vi "_시리얼_Mark10-제어 (압력설정).vi"(3 "FTS 제어 상태":T1="압력제어 시작", 4 "압력 설정(lb)":dbl=10.0 min=0.0 max=160.0 step=0.01 format="%.2f", 5 "시리얼 포트":refnum<visa-resource-name>="COM5") -> (0 "게이지 압력(lb)":dbl min=0.0 max=160.0 step=0.01 format="%.2f", 1 "통신 정상":bool=TRUE, 2 "시리얼 포트out":refnum<visa-resource-name>="COM5")   [LabVIEW 2015]
panel:
  out "미세조정 횟수":u32
  in  "속도-미세조정(mm/min)":dbl=1.0
  in  "속도-저속(mm/min)":dbl=4.0
  in  "속도-중속(mm/min)":dbl=60.0
  in  "속도-고속(mm/min)":dbl=250.0
  # "MARK10 압력 제어"
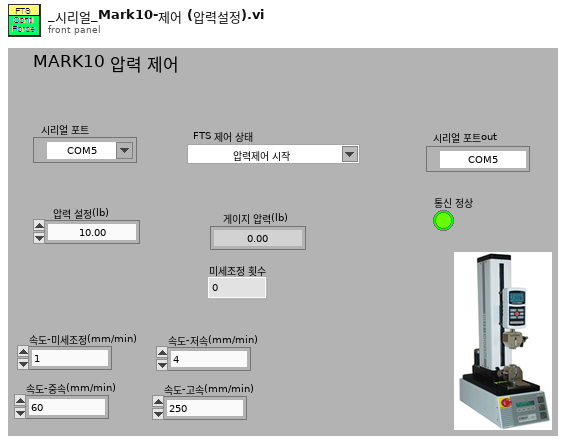
[diagram p1: front panel]
types:
  T1 = typedef "컨트롤-동작상태 FTS.ctl" = string
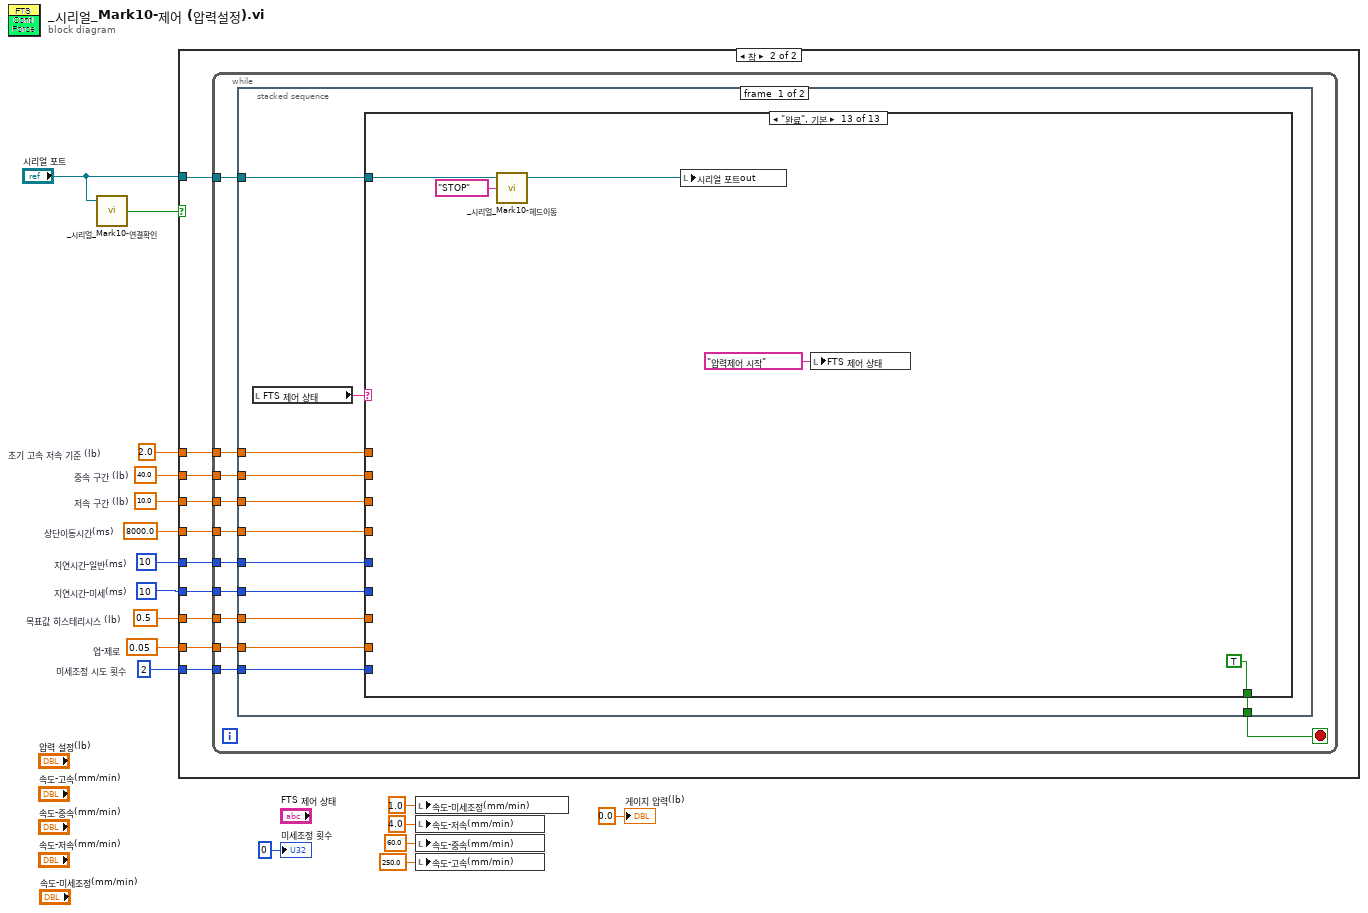
[diagram p0: block diagram]
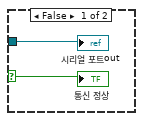
[diagram p2: hidden frame]
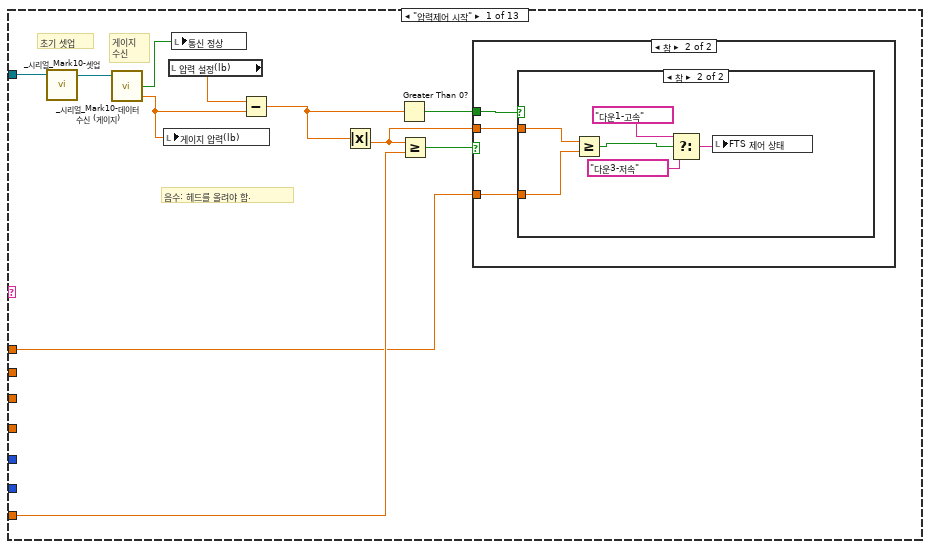
[diagram p3: hidden frame]
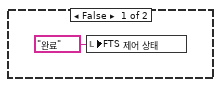
[diagram p4: hidden frame]
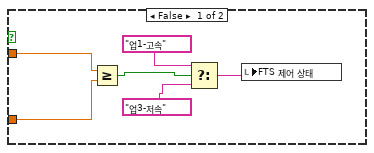
[diagram p5: hidden frame]
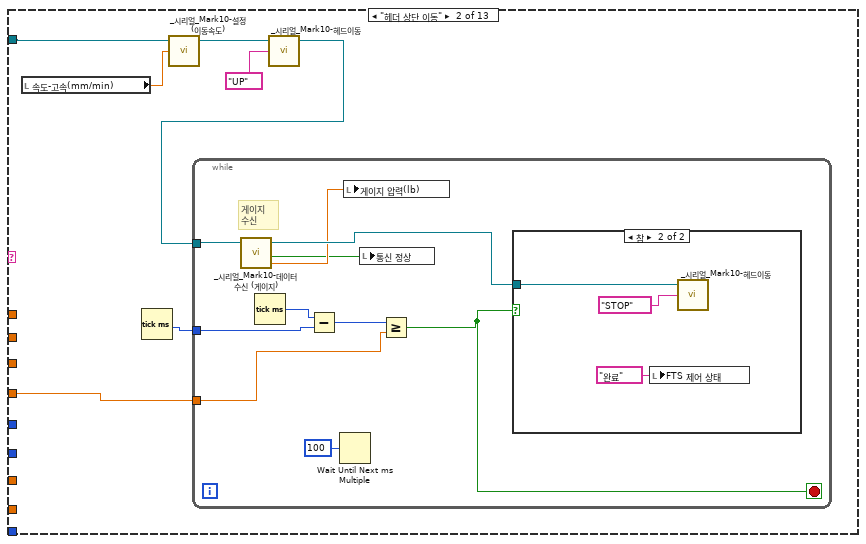
[diagram p6: hidden frame]
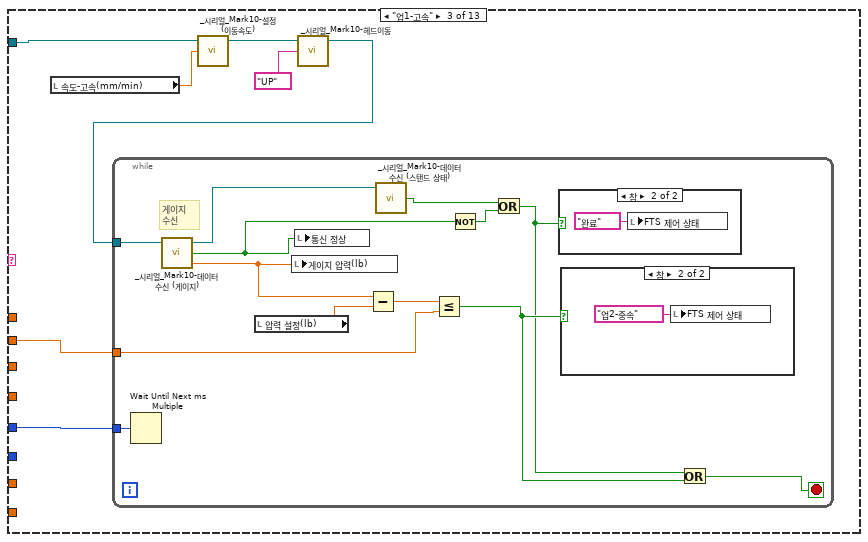
[diagram p8: hidden frame]
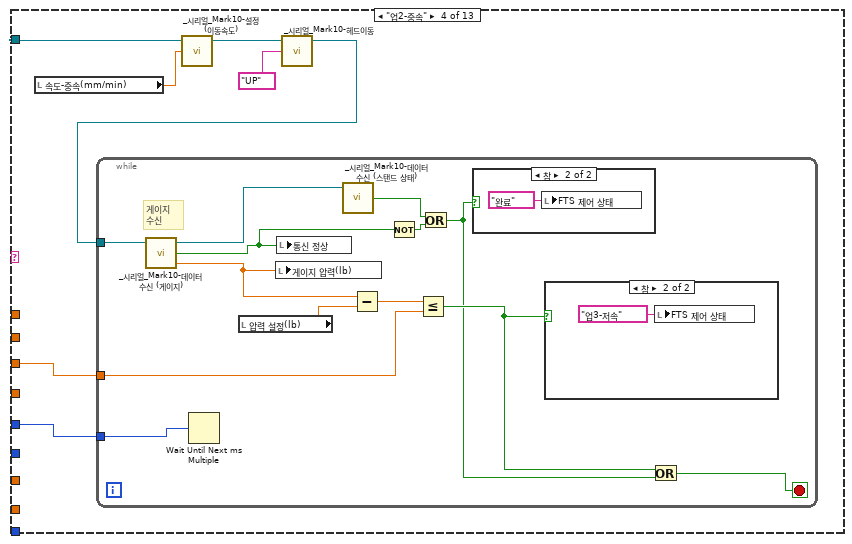
[diagram p11: hidden frame]
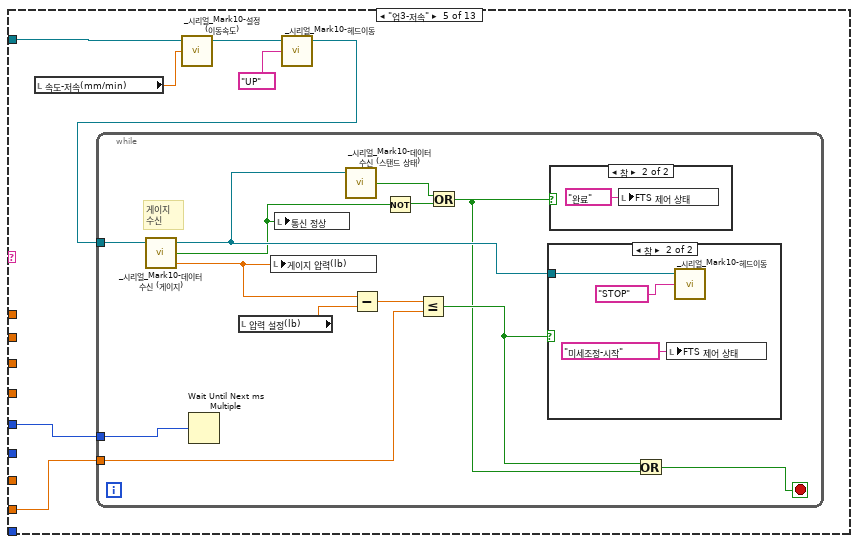
[diagram p14: hidden frame]
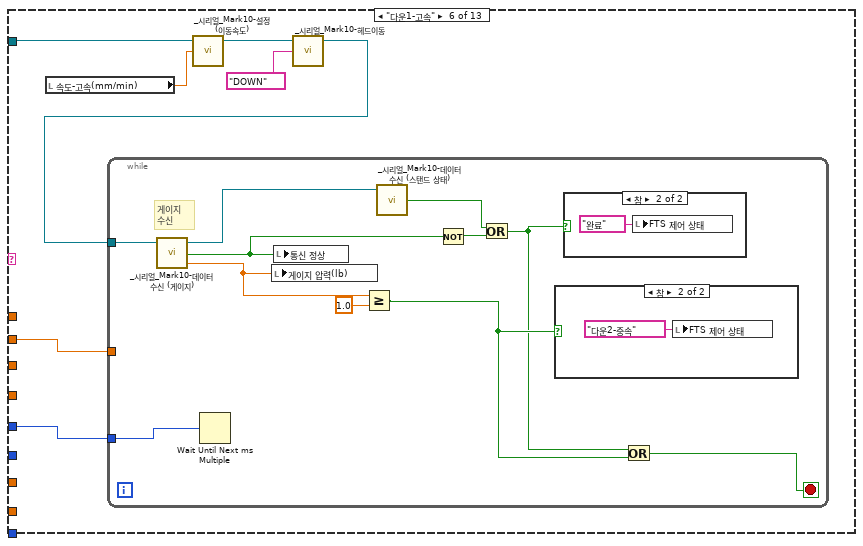
[diagram p17: hidden frame]
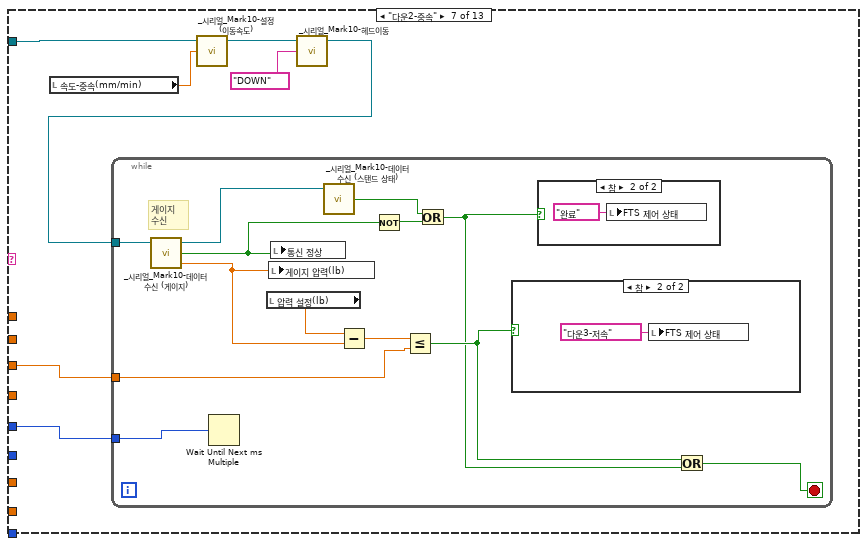
[diagram p20: hidden frame]
diagram:
  w1 = u32 2  # 미세조정 시도 횟수
  w2 = 2.0  # 초기 고속 저속 기준 (lb)
  w3 = 0.05  # 업-제로
  w5 = 0.5  # 목표값 히스테리시스 (lb)
  w10 = u32 10  # 지연시간-미세(ms)
  w11 = u32 10  # 지연시간-일반(ms)
  w12 = 8000.0  # 상단이동시간(ms)
  w13 = 10.0  # 저속 구간 (lb)
  w14 = 40.0  # 중속 구간 (lb)
  n1 = call "_시리얼_Mark10-연결확인.vi"("시리얼 포트"="시리얼 포트") -> ("수신 정상"=w15:bool)  [unwired: 3 in, 1 out]
  n2 = case shown="참" w15 {
    selector: w15 -> [w18 _]
    tunnel: "시리얼 포트" -> [w19 w29]
    tunnel: w14 -> [_ w28]
    tunnel: w13 -> [_ w27]
    tunnel: w12 -> [_ w26]
    tunnel: w11 -> [_ w25]
    tunnel: w10 -> [_ w24]
    tunnel: w5 -> [_ w23]
    tunnel: w3 -> [_ w22]
    tunnel: w2 -> [_ w21]
    tunnel: w1 -> [_ w20]
    frame False {
      "통신 정상" <- w18
      "시리얼 포트out" <- w19
    }
    frame True {
      n3 = while {
        tunnel: w29 -> [w40]
        tunnel: w28 -> [w38]
        tunnel: w27 -> [w37]
        tunnel: w26 -> [w36]
        tunnel: w25 -> [w35]
        tunnel: w24 -> [w34]
        tunnel: w23 -> [w33]
        tunnel: w22 -> [w32]
        tunnel: w21 -> [w31]
        tunnel: w20 -> [w30]
        stop <- w39 stop-if-true
        n4 = stacked-sequence {
          tunnel: w40 -> [w52 _]
          tunnel: [w50 _] -> w39
          tunnel: w38 -> [w49 _]
          tunnel: w37 -> [w48 _]
          tunnel: w36 -> [w47 _]
          tunnel: w35 -> [w46 _]
          tunnel: w34 -> [w45 _]
          tunnel: w33 -> [w44 _]
          tunnel: w32 -> [w43 _]
          tunnel: w31 -> [w42 _]
          tunnel: w30 -> [w41 _]
          frame #0 {
            n5 = local read "FTS 제어 상태"() -> (w51:T1)
            n6 = case shown="\"완료\", 기본" w51 {
              tunnel: w52 -> [w63 w82 w102 w124 w146 w173 w190 w211 w234 w262 w287 w313 w335]
              tunnel: [_ _ _ _ _ _ _ _ _ _ _ _ TRUE] -> w50
              tunnel: w49 -> [_ _ w101 _ _ w169 _ _ _ _ _ _ _]
              tunnel: w48 -> [_ _ _ w123 _ _ w189 _ _ _ _ _ _]
              tunnel: w47 -> [_ w80 _ _ _ _ _ _ _ _ _ _ _]
              tunnel: w46 -> [_ _ w100 w122 w145 w168 w188 w210 _ _ _ _ _]
              tunnel: w45 -> [_ _ _ _ _ _ _ _ _ w261 w286 _ _]
              tunnel: w44 -> [w54 _ _ _ _ _ _ _ w233 _ _ w312 _]
              tunnel: w43 -> [_ _ _ _ w144 _ _ _ _ _ w285 _ _]
              tunnel: w42 -> [w53 _ _ _ _ _ _ _ _ _ _ _ _]
              tunnel: w41 -> [_ _ _ _ _ _ _ _ _ _ _ w311 _]
              frame "압력제어 시작" {
                # "음수: 헤드를 올려야 함."
                # "게이지\n수신"
                # "초기 셋업"
                n7 = call "_시리얼_Mark10-셋업.vi"("시리얼 포트"=w63) -> ("VISA 리소스 이름 출력"=w62:refnum<visa-resource-name>)  [unwired: 4 in]
                n8 = call "_시리얼_Mark10-데이터 수신 (게이지).vi"("시리얼 포트"=w62) -> ("데이터(lb)"=w60:dbl, "수신 정상"=w55:bool)  [unwired: 2 in, 1 out]
                n9 = local write "게이지 압력(lb)"(w60) -> ()
                n10 = local read "압력 설정(lb)"() -> (w61:dbl)
                n11 = local write "통신 정상"(w55) -> ()
                n12 = Subtract(x=w61, y=w60) -> (x-y=w58:dbl)
                n13 = Absolute Value(x=w58) -> (abs(x)=w56:dbl)
                n14 = Greater Than 0?(x=w58) -> (x > 0?=w57:bool)
                n15 = Greater Or Equal?(x=w56, y=w54) -> (x >= y?=w59:bool)
                n16 = case shown="참" w59 {
                  tunnel: w57 -> [_ w67]
                  tunnel: w56 -> [_ w66]
                  tunnel: w53 -> [_ w65]
                  frame False {
                    n17 = local write "FTS 제어 상태"(T1 "완료" ("FTS 제어 상태")) -> ()
                  }
                  frame True {
                    n18 = case shown="참" w67 {
                      tunnel: w66 -> [w70 w79]
                      tunnel: w65 -> [w68 w75]
                      frame False {
                        n19 = Greater Or Equal?(x=w70, y=w68) -> (x >= y?=w73:bool)
                        n20 = Select(t=T1 "업1-고속" ("FTS 제어 상태"), s=w73, f=T1 "업3-저속" ("FTS 제어 상태")) -> (s? t:f=w69:T1)
                        n21 = local write "FTS 제어 상태"(w69) -> ()
                      }
                      frame True {
                        n22 = Greater Or Equal?(x=w79, y=w75) -> (x >= y?=w78:bool)
                        n23 = Select(t=T1 "다운1-고속" ("FTS 제어 상태"), s=w78, f=T1 "다운3-저속") -> (s? t:f=w76:T1)
                        n24 = local write "FTS 제어 상태"(w76) -> ()
                      }
                    }
                  }
                }
              }
              frame "헤더 상단 이동" {
                n25 = local read "속도-고속(mm/min)"() -> (w86:dbl)
                n26 = Tick Count (ms)() -> (millisecond timer value=w81:u32)
                n27 = call "_시리얼_Mark10-설정 (이동속도).vi"("속도(mm/min)"=w86, "시리얼 포트"=w82) -> ("VISA 리소스 이름 출력"=w84:refnum<visa-resource-name>)  [unwired: 3 in]
                n28 = call "_시리얼_Mark10-헤드이동.vi"("동작 모드"="UP", "시리얼 포트"=w84) -> ("VISA 리소스 이름 출력"=w83:refnum<visa-resource-name>)  [unwired: 3 in]
                n29 = while {
                  tunnel: w83 -> [w96]
                  tunnel: w81 -> [w91]
                  tunnel: w80 -> [w89]
                  stop <- w88 stop-if-true
                  # "게이지\n수신"
                  n30 = call "_시리얼_Mark10-데이터 수신 (게이지).vi"("시리얼 포트"=w96) -> ("데이터(lb)"=w93:dbl, "수신 정상"=w87:bool, "시리얼 포트 out"=w95:refnum<visa-resource-name>)  [unwired: 2 in]
                  n31 = Tick Count (ms)() -> (millisecond timer value=w92:u32)
                  n32 = Subtract(x=w92, y=w91) -> (x-y=w90:u32)
                  n33 = Wait Until Next ms Multiple(millisecond multiple=u32 100 ("ms 배수")) -> ()  [unwired: 1 out]
                  n34 = local write "게이지 압력(lb)"(w93) -> ()
                  n35 = local write "통신 정상"(w87) -> ()
                  n36 = Greater Or Equal?(x=w90, y=w89) -> (x >= y?=w88:bool)
                  n37 = case shown="참" w88 {
                    tunnel: w95 -> [_ w97]
                    frame False {
                    }
                    frame True {
                      n38 = local write "FTS 제어 상태"(T1 "완료" ("FTS 제어 상태")) -> ()
                      n39 = call "_시리얼_Mark10-헤드이동.vi"("동작 모드"="STOP", "시리얼 포트"=w97) -> ()  [unwired: 3 in, 1 out]
                    }
                  }
                }
              }
              frame "업1-고속" {
                n40 = local read "속도-고속(mm/min)"() -> (w106:dbl)
                n41 = call "_시리얼_Mark10-설정 (이동속도).vi"("속도(mm/min)"=w106, "시리얼 포트"=w102) -> ("VISA 리소스 이름 출력"=w104:refnum<visa-resource-name>)  [unwired: 3 in]
                n42 = call "_시리얼_Mark10-헤드이동.vi"("동작 모드"="UP", "시리얼 포트"=w104) -> ("VISA 리소스 이름 출력"=w103:refnum<visa-resource-name>)  [unwired: 3 in]
                n43 = while {
                  tunnel: w103 -> [w119]
                  tunnel: w101 -> [w115]
                  tunnel: w100 -> [w114]
                  stop <- w111 stop-if-true
                  # "게이지\n수신"
                  n44 = Wait Until Next ms Multiple(millisecond multiple=w114) -> ()  [unwired: 1 out]
                  n45 = call "_시리얼_Mark10-데이터 수신 (게이지).vi"("시리얼 포트"=w119) -> ("데이터(lb)"=w116:dbl, "수신 정상"=w107:bool, "시리얼 포트 out"=w113:refnum<visa-resource-name>)  [unwired: 2 in]
                  n46 = local read "압력 설정(lb)"() -> (w118:dbl)
                  n47 = local write "게이지 압력(lb)"(w116) -> ()
                  n48 = local write "통신 정상"(w107) -> ()
                  n49 = Subtract(x=w116, y=w118) -> (x-y=w117:dbl)
                  n50 = call "_시리얼_Mark10-데이터 수신 (스탠드 상태).vi"("시리얼 포트"=w113) -> ("모터 정지 상태"=w109:bool)  [unwired: 3 in, 1 out]
                  n51 = Less Or Equal?(x=w117, y=w115) -> (x <= y?=w112:bool)
                  n52 = Not(x=w107) -> (.not. x?=w108:bool)
                  n53 = Or(x=w109, y=w108) -> (x .or. y?=w110:bool)
                  n54 = case shown="참" w110 {
                    frame False {
                    }
                    frame True {
                      n55 = local write "FTS 제어 상태"(T1 "완료" ("FTS 제어 상태")) -> ()
                    }
                  }
                  n56 = case shown="참" w112 {
                    frame False {
                    }
                    frame True {
                      n57 = local write "FTS 제어 상태"(T1 "업2-중속" ("FTS 제어 상태")) -> ()
                    }
                  }
                  n58 = Or(x=w110, y=w112) -> (x .or. y?=w111:bool)
                }
              }
              frame "업2-중속" {
                n59 = local read "속도-중속(mm/min)"() -> (w128:dbl)
                n60 = call "_시리얼_Mark10-설정 (이동속도).vi"("속도(mm/min)"=w128, "시리얼 포트"=w124) -> ("VISA 리소스 이름 출력"=w126:refnum<visa-resource-name>)  [unwired: 3 in]
                n61 = call "_시리얼_Mark10-헤드이동.vi"("동작 모드"="UP", "시리얼 포트"=w126) -> ("VISA 리소스 이름 출력"=w125:refnum<visa-resource-name>)  [unwired: 3 in]
                n62 = while {
                  tunnel: w125 -> [w141]
                  tunnel: w123 -> [w137]
                  tunnel: w122 -> [w136]
                  stop <- w133 stop-if-true
                  # "게이지\n수신"
                  n63 = call "_시리얼_Mark10-데이터 수신 (게이지).vi"("시리얼 포트"=w141) -> ("데이터(lb)"=w138:dbl, "수신 정상"=w129:bool, "시리얼 포트 out"=w135:refnum<visa-resource-name>)  [unwired: 2 in]
                  n64 = Wait Until Next ms Multiple(millisecond multiple=w136) -> ()  [unwired: 1 out]
                  n65 = local read "압력 설정(lb)"() -> (w140:dbl)
                  n66 = local write "게이지 압력(lb)"(w138) -> ()
                  n67 = local write "통신 정상"(w129) -> ()
                  n68 = call "_시리얼_Mark10-데이터 수신 (스탠드 상태).vi"("시리얼 포트"=w135) -> ("모터 정지 상태"=w131:bool)  [unwired: 3 in, 1 out]
                  n69 = Subtract(x=w138, y=w140) -> (x-y=w139:dbl)
                  n70 = Not(x=w129) -> (.not. x?=w132:bool)
                  n71 = Less Or Equal?(x=w139, y=w137) -> (x <= y?=w134:bool)
                  n72 = Or(x=w131, y=w132) -> (x .or. y?=w130:bool)
                  n73 = case shown="참" w130 {
                    frame False {
                    }
                    frame True {
                      n74 = local write "FTS 제어 상태"(T1 "완료" ("FTS 제어 상태")) -> ()
                    }
                  }
                  n75 = case shown="참" w134 {
                    frame False {
                    }
                    frame True {
                      n76 = local write "FTS 제어 상태"(T1 "업3-저속" ("FTS 제어 상태")) -> ()
                    }
                  }
                  n77 = Or(x=w134, y=w130) -> (x .or. y?=w133:bool)
                }
              }
              frame "업3-저속" {
                n78 = local read "속도-저속(mm/min)"() -> (w150:dbl)
                n79 = call "_시리얼_Mark10-설정 (이동속도).vi"("속도(mm/min)"=w150, "시리얼 포트"=w146) -> ("VISA 리소스 이름 출력"=w148:refnum<visa-resource-name>)  [unwired: 3 in]
                n80 = call "_시리얼_Mark10-헤드이동.vi"("동작 모드"="UP", "시리얼 포트"=w148) -> ("VISA 리소스 이름 출력"=w147:refnum<visa-resource-name>)  [unwired: 3 in]
                n81 = while {
                  tunnel: w147 -> [w163]
                  tunnel: w145 -> [w159]
                  tunnel: w144 -> [w151]
                  stop <- w156 stop-if-true
                  # "게이지\n수신"
                  n82 = call "_시리얼_Mark10-데이터 수신 (게이지).vi"("시리얼 포트"=w163) -> ("데이터(lb)"=w160:dbl, "수신 정상"=w155:bool, "시리얼 포트 out"=w158:refnum<visa-resource-name>)  [unwired: 2 in]
                  n83 = Wait Until Next ms Multiple(millisecond multiple=w159) -> ()  [unwired: 1 out]
                  n84 = local read "압력 설정(lb)"() -> (w162:dbl)
                  n85 = local write "게이지 압력(lb)"(w160) -> ()
                  n86 = local write "통신 정상"(w155) -> ()
                  n87 = call "_시리얼_Mark10-데이터 수신 (스탠드 상태).vi"("시리얼 포트"=w158) -> ("모터 정지 상태"=w153:bool)  [unwired: 3 in, 1 out]
                  n88 = Subtract(x=w160, y=w162) -> (x-y=w161:dbl)
                  n89 = Not(x=w155) -> (.not. x?=w154:bool)
                  n90 = Less Or Equal?(x=w161, y=w151) -> (x <= y?=w157:bool)
                  n91 = Or(x=w153, y=w154) -> (x .or. y?=w152:bool)
                  n92 = case shown="참" w157 {
                    tunnel: w158 -> [_ w166]
                    frame False {
                    }
                    frame True {
                      n93 = local write "FTS 제어 상태"(T1 "미세조정-시작" ("FTS 제어 상태")) -> ()
                      n94 = call "_시리얼_Mark10-헤드이동.vi"("동작 모드"="STOP", "시리얼 포트"=w166) -> ()  [unwired: 3 in, 1 out]
                    }
                  }
                  n95 = case shown="참" w152 {
                    frame False {
                    }
                    frame True {
                      n96 = local write "FTS 제어 상태"(T1 "완료" ("FTS 제어 상태")) -> ()
                    }
                  }
                  n97 = Or(x=w157, y=w152) -> (x .or. y?=w156:bool)
                }
              }
              frame "다운1-고속" {
                n98 = local read "속도-고속(mm/min)"() -> (w174:dbl)
                n99 = call "_시리얼_Mark10-설정 (이동속도).vi"("속도(mm/min)"=w174, "시리얼 포트"=w173) -> ("VISA 리소스 이름 출력"=w171:refnum<visa-resource-name>)  [unwired: 3 in]
                n100 = call "_시리얼_Mark10-헤드이동.vi"("동작 모드"="DOWN", "시리얼 포트"=w171) -> ("VISA 리소스 이름 출력"=w170:refnum<visa-resource-name>)  [unwired: 3 in]
                n101 = while {
                  tunnel: w170 -> [w185]
                  tunnel: w169 -> [_]
                  tunnel: w168 -> [w182]
                  stop <- w179 stop-if-true
                  # "게이지\n수신"
                  n102 = call "_시리얼_Mark10-데이터 수신 (게이지).vi"("시리얼 포트"=w185) -> ("데이터(lb)"=w184:dbl, "수신 정상"=w178:bool, "시리얼 포트 out"=w181:refnum<visa-resource-name>)  [unwired: 2 in]
                  n103 = Wait Until Next ms Multiple(millisecond multiple=w182) -> ()  [unwired: 1 out]
                  n104 = local write "게이지 압력(lb)"(w184) -> ()
                  n105 = local write "통신 정상"(w178) -> ()
                  n106 = Greater Or Equal?(x=w184, y=1.0) -> (x >= y?=w180:bool)
                  n107 = call "_시리얼_Mark10-데이터 수신 (스탠드 상태).vi"("시리얼 포트"=w181) -> ("모터 정지 상태"=w176:bool)  [unwired: 3 in, 1 out]
                  n108 = Not(x=w178) -> (.not. x?=w177:bool)
                  n109 = Or(x=w176, y=w177) -> (x .or. y?=w175:bool)
                  n110 = case shown="참" w180 {
                    frame False {
                    }
                    frame True {
                      n111 = local write "FTS 제어 상태"(T1 "다운2-중속" ("FTS 제어 상태")) -> ()
                    }
                  }
                  n112 = case shown="참" w175 {
                    frame False {
                    }
                    frame True {
                      n113 = local write "FTS 제어 상태"(T1 "완료" ("FTS 제어 상태")) -> ()
                    }
                  }
                  n114 = Or(x=w175, y=w180) -> (x .or. y?=w179:bool)
                }
              }
              frame "다운2-중속" {
                n115 = local read "속도-중속(mm/min)"() -> (w194:dbl)
                n116 = call "_시리얼_Mark10-설정 (이동속도).vi"("속도(mm/min)"=w194, "시리얼 포트"=w190) -> ("VISA 리소스 이름 출력"=w192:refnum<visa-resource-name>)  [unwired: 3 in]
                n117 = call "_시리얼_Mark10-헤드이동.vi"("동작 모드"="DOWN", "시리얼 포트"=w192) -> ("VISA 리소스 이름 출력"=w191:refnum<visa-resource-name>)  [unwired: 3 in]
                n118 = while {
                  tunnel: w191 -> [w207]
                  tunnel: w189 -> [w203]
                  tunnel: w188 -> [w202]
                  stop <- w199 stop-if-true
                  # "게이지\n수신"
                  n119 = call "_시리얼_Mark10-데이터 수신 (게이지).vi"("시리얼 포트"=w207) -> ("데이터(lb)"=w204:dbl, "수신 정상"=w198:bool, "시리얼 포트 out"=w201:refnum<visa-resource-name>)  [unwired: 2 in]
                  n120 = Wait Until Next ms Multiple(millisecond multiple=w202) -> ()  [unwired: 1 out]
                  n121 = local read "압력 설정(lb)"() -> (w206:dbl)
                  n122 = local write "게이지 압력(lb)"(w204) -> ()
                  n123 = local write "통신 정상"(w198) -> ()
                  n124 = call "_시리얼_Mark10-데이터 수신 (스탠드 상태).vi"("시리얼 포트"=w201) -> ("모터 정지 상태"=w196:bool)  [unwired: 3 in, 1 out]
                  n125 = Subtract(x=w206, y=w204) -> (x-y=w205:dbl)
                  n126 = Not(x=w198) -> (.not. x?=w197:bool)
                  n127 = Less Or Equal?(x=w205, y=w203) -> (x <= y?=w200:bool)
                  n128 = Or(x=w196, y=w197) -> (x .or. y?=w195:bool)
                  n129 = case shown="참" w200 {
                    frame False {
                    }
                    frame True {
                      n130 = local write "FTS 제어 상태"(T1 "다운3-저속" ("FTS 제어 상태")) -> ()
                    }
                  }
                  n131 = case shown="참" w195 {
                    frame False {
                    }
                    frame True {
                      n132 = local write "FTS 제어 상태"(T1 "완료" ("FTS 제어 상태")) -> ()
                    }
                  }
                  n133 = Or(x=w200, y=w195) -> (x .or. y?=w199:bool)
                }
              }
              frame "다운3-저속" {
                n134 = local read "속도-저속(mm/min)"() -> (w215:dbl)
                n135 = call "_시리얼_Mark10-설정 (이동속도).vi"("속도(mm/min)"=w215, "시리얼 포트"=w211) -> ("VISA 리소스 이름 출력"=w213:refnum<visa-resource-name>)  [unwired: 3 in]
                n136 = call "_시리얼_Mark10-헤드이동.vi"("동작 모드"="DOWN", "시리얼 포트"=w213) -> ("VISA 리소스 이름 출력"=w212:refnum<visa-resource-name>)  [unwired: 3 in]
                n137 = while {
                  tunnel: w212 -> [w228]
                  tunnel: w210 -> [w224]
                  stop <- w222 stop-if-true
                  # "게이지\n수신"
                  n138 = call "_시리얼_Mark10-데이터 수신 (게이지).vi"("시리얼 포트"=w228) -> ("데이터(lb)"=w225:dbl, "수신 정상"=w216:bool, "시리얼 포트 out"=w221:refnum<visa-resource-name>)  [unwired: 2 in]
                  n139 = Wait Until Next ms Multiple(millisecond multiple=w224) -> ()  [unwired: 1 out]
                  n140 = local write "통신 정상"(w216) -> ()
                  n141 = local read "압력 설정(lb)"() -> (w227:dbl)
                  n142 = local write "게이지 압력(lb)"(w225) -> ()
                  n143 = Subtract(x=w227, y=w225) -> (x-y=w226:dbl)
                  n144 = call "_시리얼_Mark10-데이터 수신 (스탠드 상태).vi"("시리얼 포트"=w221) -> ("모터 정지 상태"=w219:bool, "시리얼 포트 out"=w220:refnum<visa-resource-name>)  [unwired: 3 in]
                  n145 = Less Or Equal To 0?(x=w226) -> (x <= 0?=w223:bool)
                  n146 = Not(x=w216) -> (.not. x?=w218:bool)
                  n147 = Or(x=w219, y=w218) -> (x .or. y?=w217:bool)
                  n148 = case shown="참" w223 {
                    tunnel: w220 -> [_ w231]
                    frame False {
                    }
                    frame True {
                      n149 = local write "FTS 제어 상태"(T1 "미세조정-시작" ("FTS 제어 상태")) -> ()
                      n150 = call "_시리얼_Mark10-헤드이동.vi"("동작 모드"="STOP", "시리얼 포트"=w231) -> ()  [unwired: 3 in, 1 out]
                    }
                  }
                  n151 = case shown="참" w217 {
                    frame False {
                    }
                    frame True {
                      n152 = local write "FTS 제어 상태"(T1 "완료" ("FTS 제어 상태")) -> ()
                    }
                  }
                  n153 = Or(x=w223, y=w217) -> (x .or. y?=w222:bool)
                }
              }
              frame "미세조정-시작" {
                n154 = stacked-sequence {
                  tunnel: w234 -> [w237 w255]
                  tunnel: w233 -> [_ w252]
                  frame #0 {
                    w235 = u32 500  # 타임아웃(ms)
                    # "압력 안정 될때가지 대기"
                    n155 = Tick Count (ms)() -> (millisecond timer value=w236:u32)
                    n156 = while {
                      tunnel: w237 -> [w246]
                      tunnel: w236 -> [w242]
                      tunnel: w235 -> [w240]
                      stop <- w239 stop-if-true
                      # "게이지\n수신"
                      n157 = call "_시리얼_Mark10-데이터 수신 (게이지).vi"("시리얼 포트"=w246) -> ("데이터(lb)"=w244:dbl, "수신 정상"=w238:bool)  [unwired: 2 in, 1 out]
                      n158 = Tick Count (ms)() -> (millisecond timer value=w243:u32)
                      n159 = Subtract(x=w243, y=w242) -> (x-y=w241:u32)
                      n160 = local write "게이지 압력(lb)"(w244) -> ()
                      n161 = local write "통신 정상"(w238) -> ()
                      n162 = Wait Until Next ms Multiple(millisecond multiple=u32 50 ("ms 배수")) -> ()  [unwired: 1 out]
                      n163 = Greater Or Equal?(x=w241, y=w240) -> (x >= y?=w239:bool)
                    }
                  }
                  frame #1 {
                    # "음수: 헤드를 올려야 함."
                    # "게이지\n수신"
                    n164 = call "_시리얼_Mark10-데이터 수신 (게이지).vi"("시리얼 포트"=w255) -> ("데이터(lb)"=w256:dbl, "수신 정상"=w254:bool)  [unwired: 2 in, 1 out]
                    n165 = local write "게이지 압력(lb)"(w256) -> ()
                    n166 = local read "압력 설정(lb)"() -> (w257:dbl)
                    n167 = local write "통신 정상"(w254) -> ()
                    n168 = Subtract(x=w257, y=w256) -> (x-y=w253:dbl)
                    n169 = Multiply(x=w252, y=-1.0) -> (x*y=w251:dbl)
                    n170 = Greater Or Equal?(x=w253, y=w252) -> (x >= y?=w248:bool)
                    n171 = Less Or Equal?(x=w253, y=w251) -> (x <= y?=w249:bool)
                    n172 = Or(x=w249, y=w248) -> (x .or. y?=w247:bool)
                    n173 = case shown="참" w248 {
                      frame False {
                      }
                      frame True {
                        n174 = local write "FTS 제어 상태"(T1 "미세조정-다운" ("FTS 제어 상태")) -> ()
                      }
                    }
                    n175 = case shown="참" w249 {
                      frame False {
                      }
                      frame True {
                        n176 = local write "FTS 제어 상태"(T1 "미세조정-업" ("FTS 제어 상태")) -> ()
                      }
                    }
                    n177 = case shown="거짓" w247 {
                      frame False {
                        n178 = local write "FTS 제어 상태"(T1 "미세조정-종료" ("FTS 제어 상태")) -> ()
                      }
                      frame True {
                      }
                    }
                  }
                }
              }
              frame "미세조정-다운" {
                n179 = local read "속도-미세조정(mm/min)"() -> (w266:dbl)
                n180 = call "_시리얼_Mark10-설정 (이동속도).vi"("속도(mm/min)"=w266, "시리얼 포트"=w262) -> ("VISA 리소스 이름 출력"=w264:refnum<visa-resource-name>)  [unwired: 3 in]
                n181 = call "_시리얼_Mark10-헤드이동.vi"("동작 모드"="DOWN", "시리얼 포트"=w264) -> ("VISA 리소스 이름 출력"=w263:refnum<visa-resource-name>)  [unwired: 3 in]
                n182 = while {
                  tunnel: w263 -> [w279]
                  tunnel: w261 -> [w273]
                  stop <- w274 stop-if-true
                  # "게이지\n수신"
                  n183 = call "_시리얼_Mark10-데이터 수신 (게이지).vi"("시리얼 포트"=w279) -> ("데이터(lb)"=w276:dbl, "수신 정상"=w267:bool, "시리얼 포트 out"=w272:refnum<visa-resource-name>)  [unwired: 2 in]
                  n184 = local write "통신 정상"(w267) -> ()
                  n185 = local read "압력 설정(lb)"() -> (w278:dbl)
                  n186 = local write "게이지 압력(lb)"(w276) -> ()
                  n187 = call "_시리얼_Mark10-데이터 수신 (스탠드 상태).vi"("시리얼 포트"=w272) -> ("모터 정지 상태"=w269:bool, "시리얼 포트 out"=w271:refnum<visa-resource-name>)  [unwired: 3 in]
                  n188 = Subtract(x=w278, y=w276) -> (x-y=w277:dbl)
                  n189 = Not(x=w267) -> (.not. x?=w270:bool)
                  n190 = Less Or Equal To 0?(x=w277) -> (x <= 0?=w275:bool)
                  n191 = Or(x=w269, y=w270) -> (x .or. y?=w268:bool)
                  n192 = case shown="참" w275 {
                    tunnel: w271 -> [_ w283]
                    tunnel: w273 -> [w281 _]
                    frame False {
                      n193 = Wait Until Next ms Multiple(millisecond multiple=w281) -> ()  [unwired: 1 out]
                    }
                    frame True {
                      n194 = local write "FTS 제어 상태"(T1 "미세조정-종료" ("FTS 제어 상태")) -> ()
                      n195 = call "_시리얼_Mark10-헤드이동.vi"("동작 모드"="STOP", "시리얼 포트"=w283) -> ()  [unwired: 3 in, 1 out]
                    }
                  }
                  n196 = case shown="참" w268 {
                    frame False {
                    }
                    frame True {
                      n197 = local write "FTS 제어 상태"(T1 "완료" ("FTS 제어 상태")) -> ()
                    }
                  }
                  n198 = Or(x=w275, y=w268) -> (x .or. y?=w274:bool)
                }
              }
              frame "미세조정-업" {
                n199 = local read "속도-저속(mm/min)"() -> (w291:dbl)
                n200 = call "_시리얼_Mark10-설정 (이동속도).vi"("속도(mm/min)"=w291, "시리얼 포트"=w287) -> ("VISA 리소스 이름 출력"=w289:refnum<visa-resource-name>)  [unwired: 3 in]
                n201 = call "_시리얼_Mark10-헤드이동.vi"("동작 모드"="UP", "시리얼 포트"=w289) -> ("VISA 리소스 이름 출력"=w288:refnum<visa-resource-name>)  [unwired: 3 in]
                n202 = while {
                  tunnel: w288 -> [w305]
                  tunnel: w286 -> [w299]
                  tunnel: w285 -> [w292]
                  stop <- w300 stop-if-true
                  # "게이지\n수신"
                  n203 = call "_시리얼_Mark10-데이터 수신 (게이지).vi"("시리얼 포트"=w305) -> ("데이터(lb)"=w302:dbl, "수신 정상"=w294:bool, "시리얼 포트 out"=w298:refnum<visa-resource-name>)  [unwired: 2 in]
                  n204 = local read "압력 설정(lb)"() -> (w304:dbl)
                  n205 = local write "게이지 압력(lb)"(w302) -> ()
                  n206 = local write "통신 정상"(w294) -> ()
                  n207 = call "_시리얼_Mark10-데이터 수신 (스탠드 상태).vi"("시리얼 포트"=w298) -> ("모터 정지 상태"=w296:bool, "시리얼 포트 out"=w297:refnum<visa-resource-name>)  [unwired: 3 in]
                  n208 = Subtract(x=w302, y=w304) -> (x-y=w303:dbl)
                  n209 = Not(x=w294) -> (.not. x?=w295:bool)
                  n210 = Less Or Equal?(x=w303, y=w292) -> (x <= y?=w301:bool)
                  n211 = Or(x=w296, y=w295) -> (x .or. y?=w293:bool)
                  n212 = case shown="참" w293 {
                    frame False {
                    }
                    frame True {
                      n213 = local write "FTS 제어 상태"(T1 "완료" ("FTS 제어 상태")) -> ()
                    }
                  }
                  n214 = case shown="참" w301 {
                    tunnel: w297 -> [_ w309]
                    tunnel: w299 -> [w307 _]
                    frame False {
                      n215 = Wait Until Next ms Multiple(millisecond multiple=w307) -> ()  [unwired: 1 out]
                    }
                    frame True {
                      n216 = local write "FTS 제어 상태"(T1 "미세조정-종료" ("FTS 제어 상태")) -> ()
                      n217 = call "_시리얼_Mark10-헤드이동.vi"("동작 모드"="STOP", "시리얼 포트"=w309) -> ()  [unwired: 3 in, 1 out]
                    }
                  }
                  n218 = Or(x=w301, y=w293) -> (x .or. y?=w300:bool)
                }
              }
              frame "미세조정-종료" {
                n219 = stacked-sequence {
                  tunnel: w313 -> [_ w318]
                  tunnel: w312 -> [_ w316]
                  tunnel: w311 -> [_ w315]
                  frame #0 {
                    n220 = Wait Until Next ms Multiple(millisecond multiple=u32 1000 ("ms 배수")) -> ()  [unwired: 1 out]
                  }
                  frame #1 {
                    # "게이지\n수신"
                    n221 = call "_시리얼_Mark10-데이터 수신 (게이지).vi"("시리얼 포트"=w318) -> ("데이터(lb)"=w322:dbl, "수신 정상"=w317:bool)  [unwired: 2 in, 1 out]
                    n222 = local write "게이지 압력(lb)"(w322) -> ()
                    n223 = local read "압력 설정(lb)"() -> (w323:dbl)
                    n224 = local write "통신 정상"(w317) -> ()
                    n225 = Subtract(x=w323, y=w322) -> (x-y=w320:dbl)
                    n226 = Absolute Value(x=w320) -> (abs(x)=w319:dbl)
                    n227 = Greater Or Equal?(x=w319, y=w316) -> (x >= y?=w321:bool)
                    n228 = case shown="거짓" w321 {
                      tunnel: w315 -> [w324 _]
                      frame False {
                        # "목표치 도달"
                        n229 = local read "미세조정 횟수"() -> (w327:u32)
                        n230 = Increment(x=w327) -> (x+1=w326:u32)
                        n231 = Greater Or Equal?(x=w326, y=w324) -> (x >= y?=w325:bool)
                        n232 = case shown="거짓" w325 {
                          frame False {
                            n233 = local write "FTS 제어 상태"(T1 "미세조정-시작" ("FTS 제어 상태")) -> ()
                          }
                          frame True {
                            n234 = local write "FTS 제어 상태"(T1 "완료" ("FTS 제어 상태")) -> ()
                          }
                        }
                        n235 = local write "미세조정 횟수"(w326) -> ()
                      }
                      frame True {
                        n236 = local write "미세조정 횟수"(u32 0 ("미세조정 횟수")) -> ()
                        n237 = local write "FTS 제어 상태"(T1 "미세조정-시작" ("FTS 제어 상태")) -> ()
                      }
                    }
                  }
                }
              }
              frame "완료", Default {
                n238 = call "_시리얼_Mark10-헤드이동.vi"("동작 모드"="STOP", "시리얼 포트"=w335) -> ("VISA 리소스 이름 출력"=w332:refnum<visa-resource-name>)  [unwired: 3 in]
                n239 = local write "시리얼 포트out"(w332) -> ()
                n240 = local write "FTS 제어 상태"(T1 "압력제어 시작" ("FTS 제어 상태")) -> ()
              }
            }
          }
          frame #1 {
            n241 = local read "통신 정상"() -> (w337:bool)
            n242 = case shown="거짓" w337 {
              frame False {
                # "BLE 버퍼 클리어"
                # "통신 에러"
                n243 = local write "FTS 제어 상태"(T1 "완료" ("FTS 제어 상태")) -> ()
                n244 = call "SUB-BLE Rx data Clear.vi"() -> ()  [unwired: 6 in]
              }
              frame True {
              }
            }
          }
        }
      }
    }
  }
  n245 = local write "속도-미세조정(mm/min)"(1.0 ("속도-미세조정(mm/min)")) -> ()
  n246 = local write "속도-저속(mm/min)"(4.0 ("속도-저속(mm/min)")) -> ()
  n247 = local write "속도-중속(mm/min)"(60.0 ("속도-중속(mm/min)")) -> ()
  n248 = local write "속도-고속(mm/min)"(250.0 ("속도-고속(mm/min)")) -> ()
  "게이지 압력(lb)" <- 0.0 ("게이지 압력(lb)")
  "미세조정 횟수" <- u32 0 ("지연시간-미세(ms)")
